vi "MenuTab DEMO.vi"() -> ()   [LabVIEW 2020]
uses:
  QMenu Class/Active Event Data.ctl
  QMenu Class/Button Attribute.ctl
  QMenu Class/QMenu Class.lvclass/QMenu Class.ctl
  QMenu Class/Read Notifier User Event.vi
  QMenu Class/Write Close Timeout.vi
  QMenu Class/Write Drag Timeout.vi
  QMenu Class/QMenu Class.lvclass
panel:
  in  "Label":string[](array[string])
  in  "Close BTN":bool
  out "Active Event Data":T1
  in  "Get Active Index":bool
  out "Drag Label":string
  out "Drag Index":i32
  out "Close Label":string
  out "Close Index":i32
  out "Iteration":i32=-1
  out "Select Label":string
  out "Select Index":i32
  out "2D Picture":picture
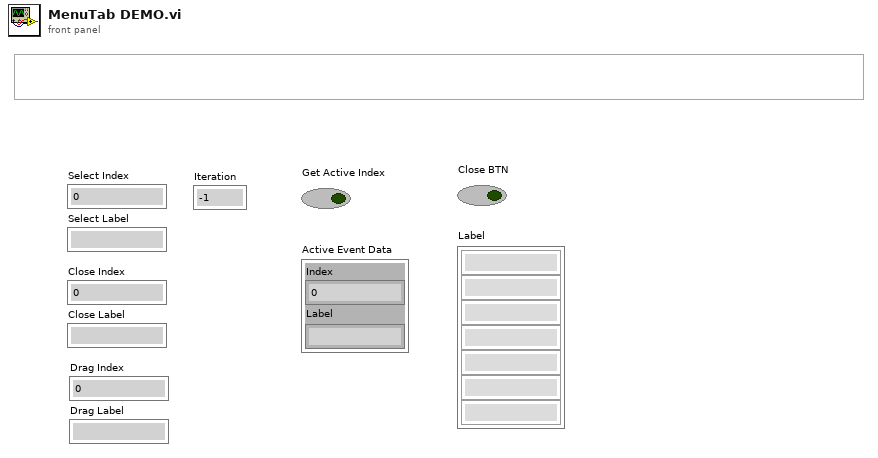
[diagram p1: front panel]
types:
  T1 = typedef "QTab.lvlib/QMenu Class.lvclass/Active Event Data.ctl" = cluster{"Index":i32, "Label":string}
  T2 = typedef "QTab.lvlib/QMenu Class.lvclass/Button Attribute.ctl" = cluster{"Label":string, "Button Text":string, "Closable":bool, "Draggable":bool}
  T3 = typedef "QTab.lvlib/QMenu Class.lvclass/Notifier User Event.ctl" = cluster{"Active User Event":refnum<user-event>, "Close User Event":refnum<user-event>, "Drag User Event":refnum<user-event>}
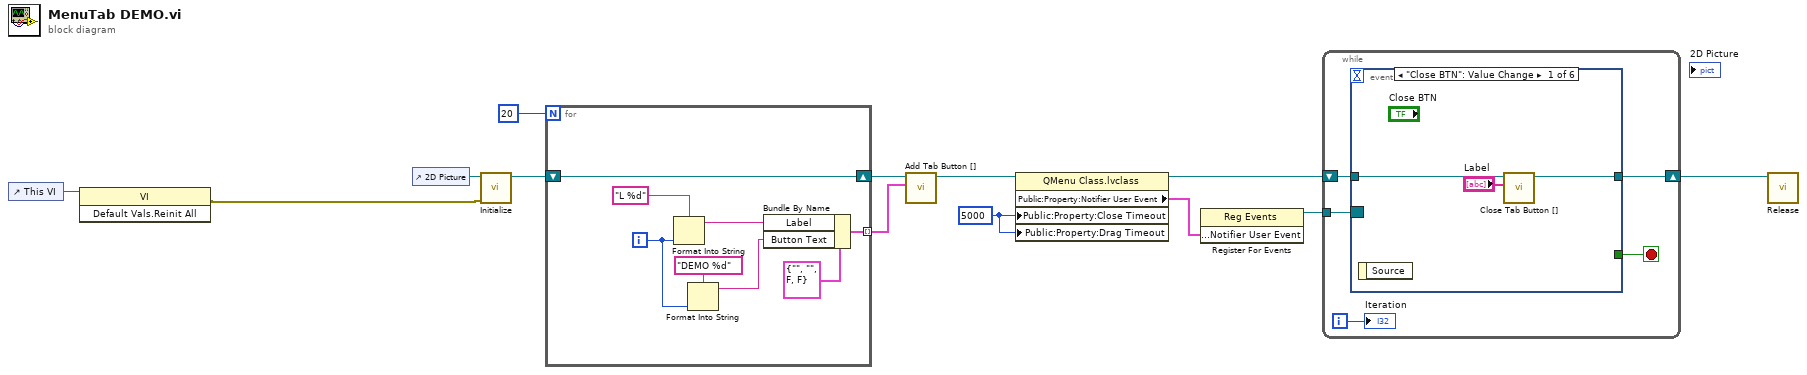
[diagram p0: block diagram]
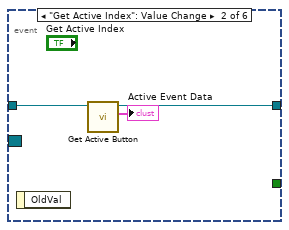
[diagram p2: hidden frame]
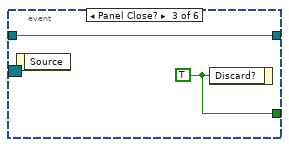
[diagram p3: hidden frame]
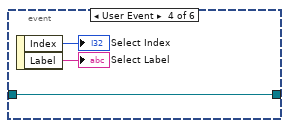
[diagram p4: hidden frame]
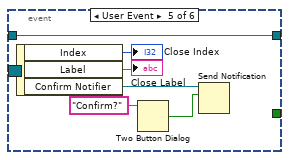
[diagram p5: hidden frame]
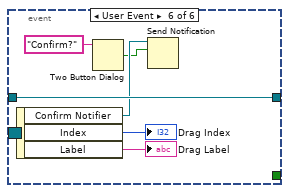
[diagram p6: hidden frame]
diagram:
  w5 = 5000 ("Close Timeout")
  n1 = control-ref of="This VI"() -> (w7:refnum<vi>)
  n2 = invoke class="VI" method="Default Vals.Reinit All"(reference=w7) -> (error out=w1:errorcluster)  [unwired: 2 in, 2 out]
  n3 = control-ref of="2D Picture"() -> (w13:refnum<vi>)
  n4 = call "Initialize.vi"("error in (no error)"=w1, "Pict Refnum"=w13) -> ("QMenu Class out"=w6:refnum<class "QMenu Class.lvclass">)  [unwired: 8 in, 1 out]
  n5 = for {
    N: 20 -> [_]
    shift-right: [w15] -> w4
    shift-left: w6 -> [w15]
    tunnel: [w14] -> w2 mode=indexing
    i -> [w21]
    n6 = Format Into String(format string="L %d", w21) -> (resulting string=w17:string)  [unwired: 2 in, 1 out]
    n7 = Format Into String(format string="DEMO %d", w21) -> (resulting string=w16:string)  [unwired: 2 in, 1 out]
    n8 = Bundle By Name(cluster=T2 {"Label"="", "Button Text"="", "Closable"=FALSE, "Draggable"=FALSE} ("Button Attribute"), "Label"=w17, "Button Text"=w16) -> (w14:T2)
  }
  n9 = call "Add Tab Button [].vi"("Button Attribute []"=w2, "QMenu Class in"=w4) -> ("QMenu Class out"=w3:refnum<class "QMenu Class.lvclass">)  [unwired: 8 in, 1 out]
  n10 = property class="QMenu Class.lvclass"(reference=w3, "Public:Property:Close Timeout"=w5, "Public:Property:Drag Timeout"=w5) -> (reference out=w10:refnum<class "QMenu Class.lvclass">, "Public:Property:Notifier User Event"=w8:T3)  [unwired: 1 in, 1 out]
  n11 = register-events(w8) -> (reference out=w9:refnum<event-registration>)  [unwired: 2 in, 1 out]
  n12 = while {
    tunnel: w9 -> [w24]
    shift-right: [w26] -> w12
    shift-left: w10 -> [w25]
    i -> [w22]
    stop <- w23 stop-if-true
    n13 = event shown="[0] \"Close BTN\": Value Change" {
      selector: w24 -> [_ _ _ _ _ _]
      dyn-events: _ -> [_ _ _ _ _ _]
      timeout: _ -> [_ _ _ _ _ _]
      tunnel: w25 -> [w29 w31 w34 w37 w40 w49]
      tunnel: [w28 w32 w34 w37 w40 w49] -> w26
      tunnel: [_ _ w33 _ _ _] -> w23
      event "Close BTN": Value Change {
        n14 = event-data() -> ()  [unwired: 1 in, 1 out]
        n15 = call "Close Tab Button [].vi"("Label"="Label", "QMenu Class in"=w29) -> ("QMenu Class out"=w28:refnum<class "QMenu Class.lvclass">)  [unwired: 8 in, 1 out]
      }
      event "Get Active Index": Value Change {
        n16 = event-data() -> ()  [unwired: 1 in, 1 out]
        n17 = call "Get Active Button.vi"("QMenu Class in"=w31) -> ("Active Event Data"=→"Active Event Data":T1, "QMenu Class out"=w32:refnum<class "QMenu Class.lvclass">)  [unwired: 8 in, 1 out]
      }
      event Panel Close? {
        w33 = TRUE ("Discard?")
        n18 = event-data() -> ()  [unwired: 1 in, 1 out]
        n19 = event-data("Discard?"=w33) -> ()  [unwired: 1 in, 1 out]
      }
      event User Event {
        n20 = event-data() -> ("Index"=→"Select Index":i32, "Label"=→"Select Label":string)  [unwired: 1 in]
      }
      event User Event {
        n21 = event-data() -> ("Index"=→"Close Index":i32, "Label"=→"Close Label":string, "Confirm Notifier"=w41:refnum<notifier>)  [unwired: 1 in]
        n22 = Two Button Dialog(message="Confirm?") -> (T button?=w39:bool)  [unwired: 2 in]
        n23 = Send Notification(notification=w39, notifier=w41) -> ()  [unwired: 1 in, 2 out]
      }
      event User Event {
        n24 = event-data() -> ("Confirm Notifier"=w46:refnum<notifier>, "Index"=→"Drag Index":i32, "Label"=→"Drag Label":string)  [unwired: 1 in]
        n25 = Two Button Dialog(message="Confirm?") -> (T button?=w44:bool)  [unwired: 2 in]
        n26 = Send Notification(notification=w44, notifier=w46) -> ()  [unwired: 1 in, 2 out]
      }
    }
    "Iteration" <- w22
  }
  n27 = call "Release.vi"("QMenu Class in"=w12) -> ()  [unwired: 10 in, 1 out]
